vi "mohlat.vi"() -> ()   [LabVIEW 2017]
uses:
  <vilib>/Instr/_visa.llb/VISA Configure Serial Port (Instr).vi
  <vilib>/Utility/file.llb/Read Delimited Spreadsheet (string).vi
  <vilib>/Utility/file.llb/Write Delimited Spreadsheet (string).vi
panel:
  in  "pass":string="1234"
  out "number of users":i32
  in  "new pass":string caption="please enter new password"
  out "array w/ subset deleted":i32[](array[numeric])
  out "Array":i32[](array[numeric])
  out "subarray":string[][](array[string])
  out "min value":i32
  out "max value":i32
  out "SERIAL ID":string
  out "FULL NAME":string
  out "picture3":picture
  out "concatenated string":string
  out "appended array 4":string[](array[string])
  out "appended array 3":string[][](array[string])
  out "sabte tarikh":string[][](array[string])
  out "payam":string
  out "matrix of the data":string[][](array[string])
  in  "file path (text format)":path
  out "appended array 2":string[][](array[string])
  out "output array":string[](array[string])
  out "data base":string[][](array[string])
  out "appended array":string[](array[string])
  out "massage":string
  in  "Cluster":T1
  in  "Boolean":bool
  in  "Combo Box":string(combo)
  in  "password":bool
  in  "password:":string caption="enter password"
  out "PASSWORD MASSAGE":string
  out "error out":errorcluster
  in  "VISA resource name":refnum<visa-resource-name>
  out "read buffer":string
  in  "stop":bool
  in  "setting":bool
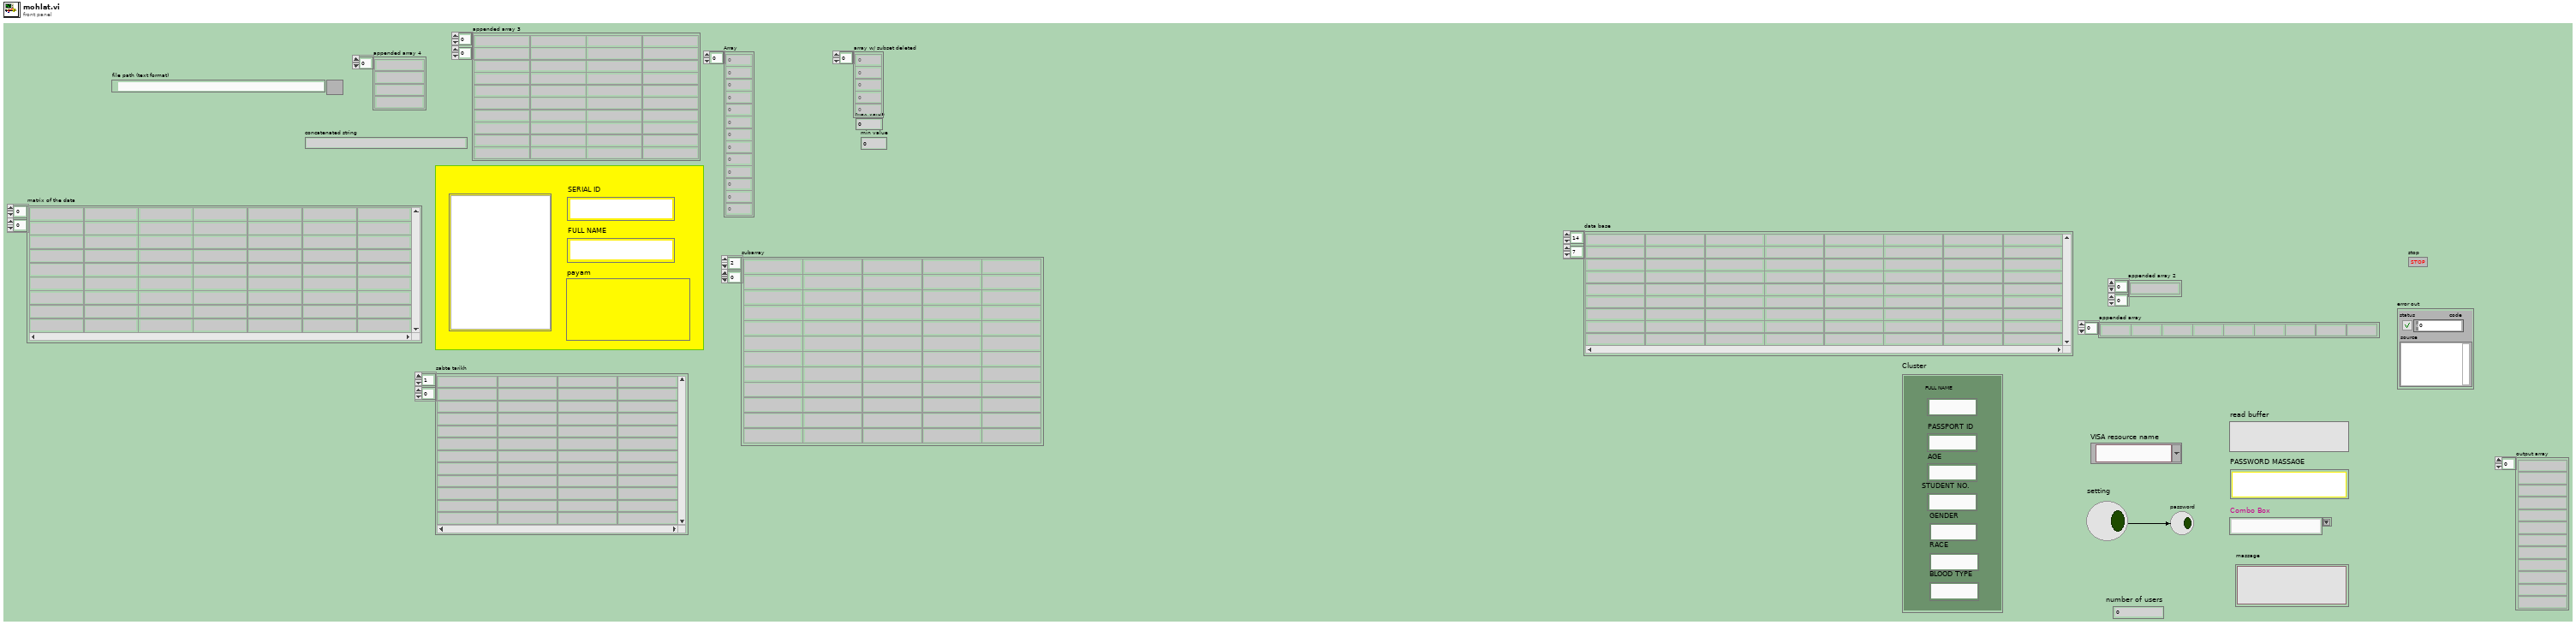
[diagram p1: front panel]
types:
  T1 = cluster{"FULL NAME":string, "PASSPORT ID":string, "AGE":string, "STUDENT NO.":string, "GENDER":string, "RACE":string, "BLOOD TYPE":string}
  T2 = cluster{"all rows[0]":string, "all rows[1]":string, "all rows[2]":string, "all rows[3]":string, "all rows[4]":string, "all rows[5]":string, "all rows[6]":string, "all rows[7]":string, "all rows[8]":string}
  T3 = typedef "imagedata.ctl" = cluster{"image type":i32, "image depth":i32, "image":u8[], "mask":u8[], "colors":u32[], "Rectangle":cluster{"left":i16, "top":i16, "right":i16, "bottom":i16}}
  T4 = cluster{string, string, string, string, string, string, string}
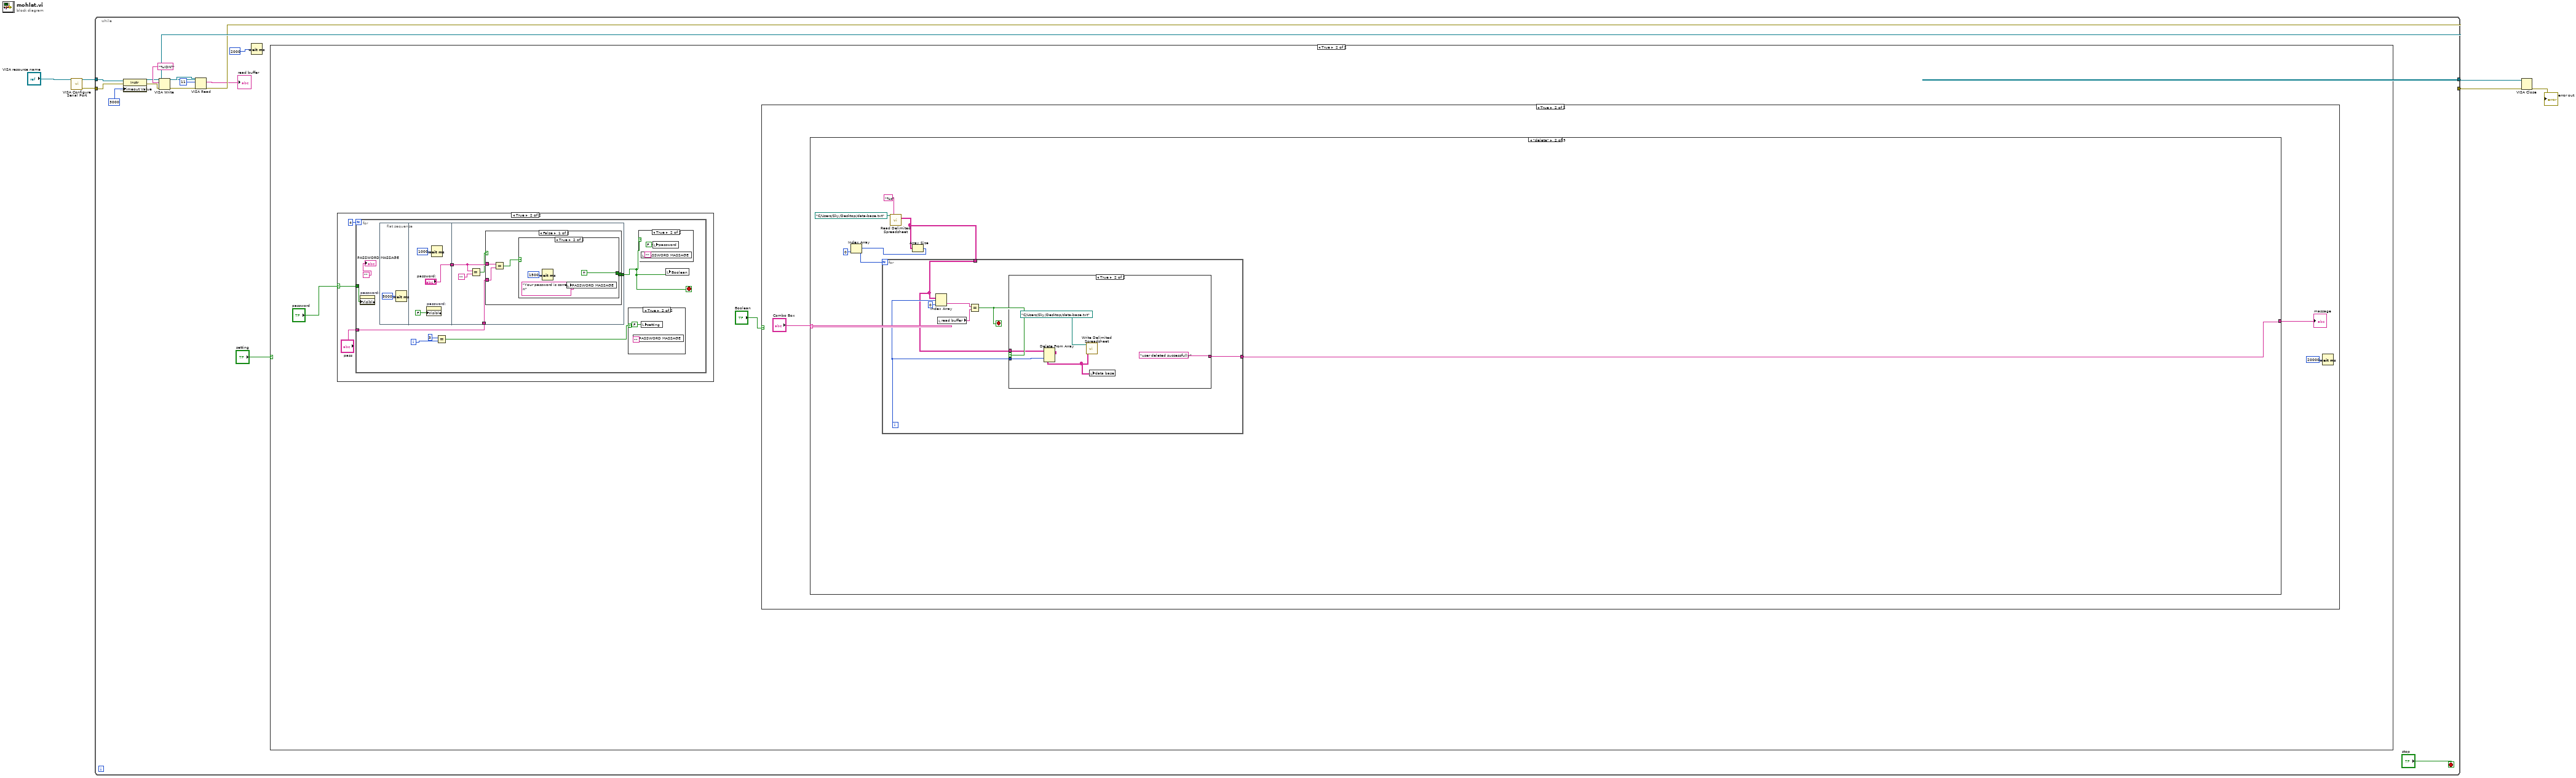
[diagram p0: block diagram]
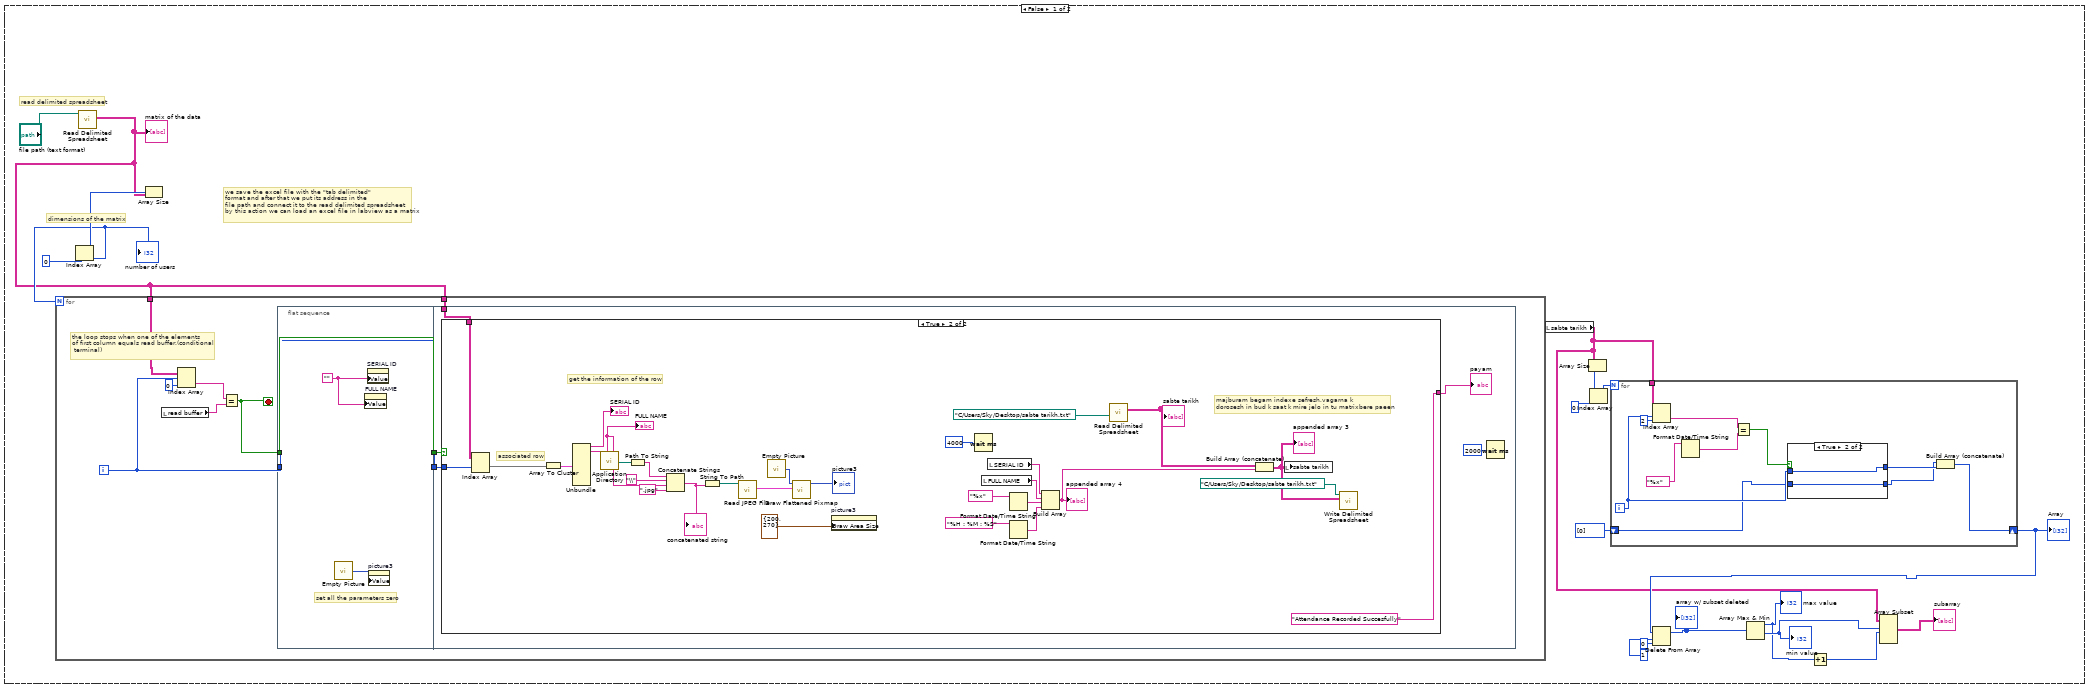
[diagram p2: hidden frame]
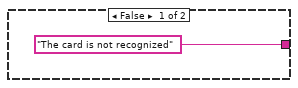
[diagram p4: hidden frame]
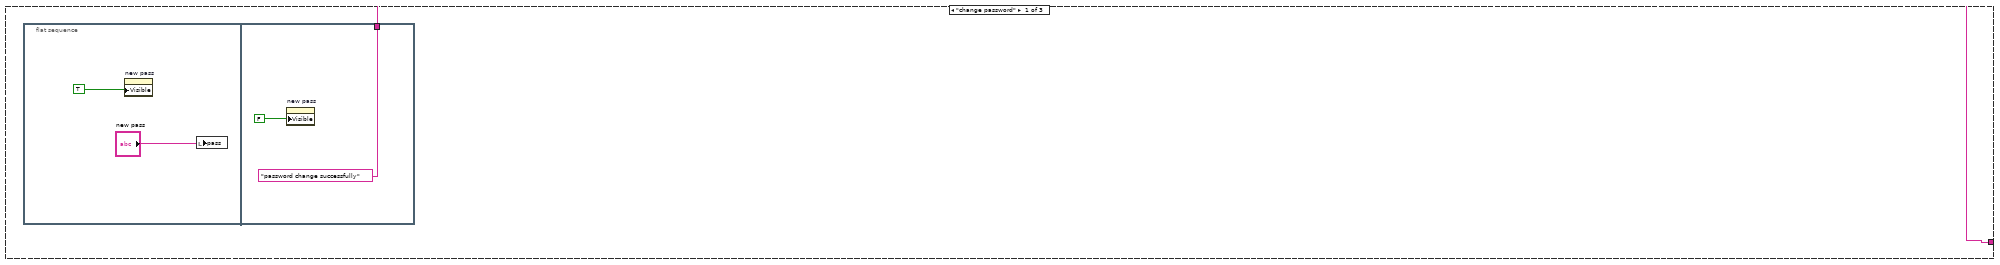
[diagram p6: hidden frame]
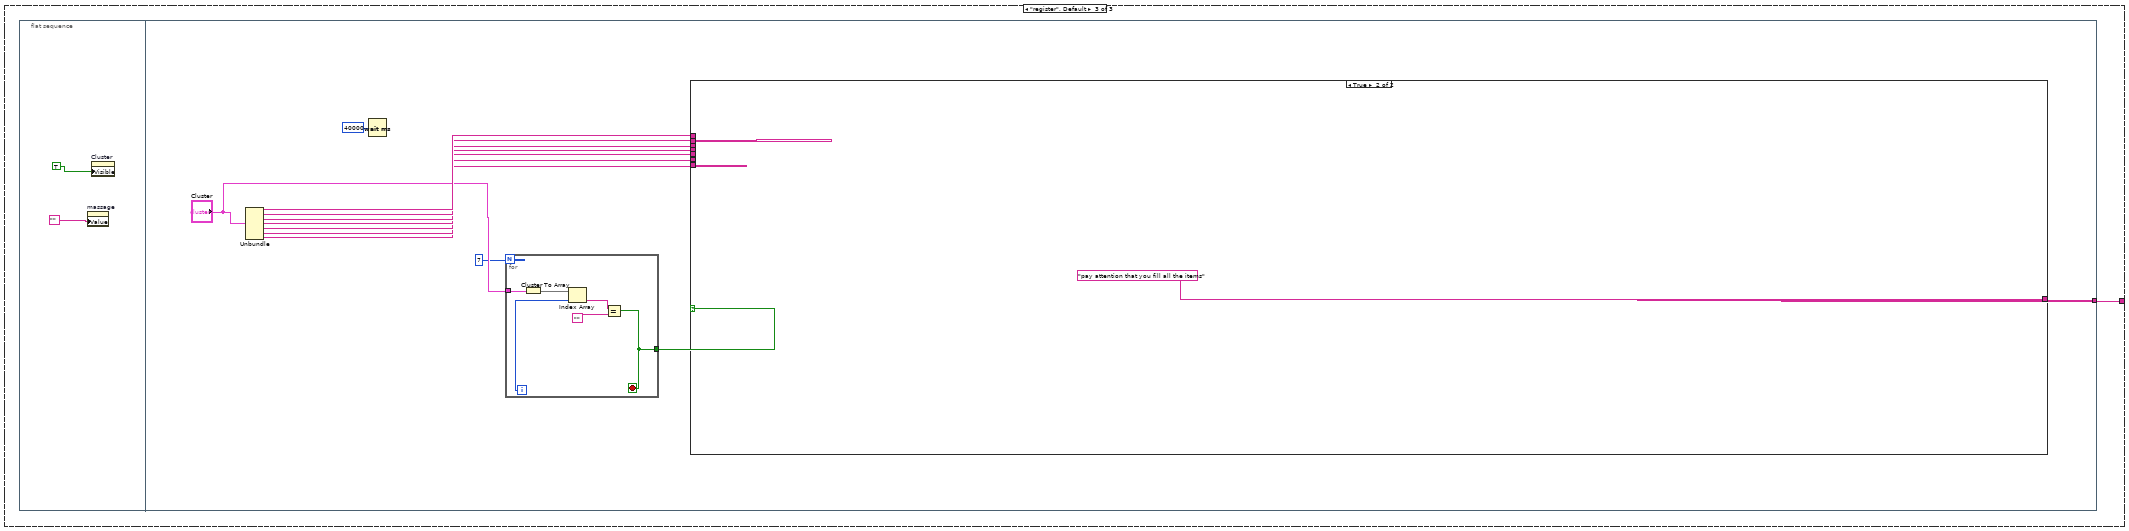
[diagram p8: hidden frame]
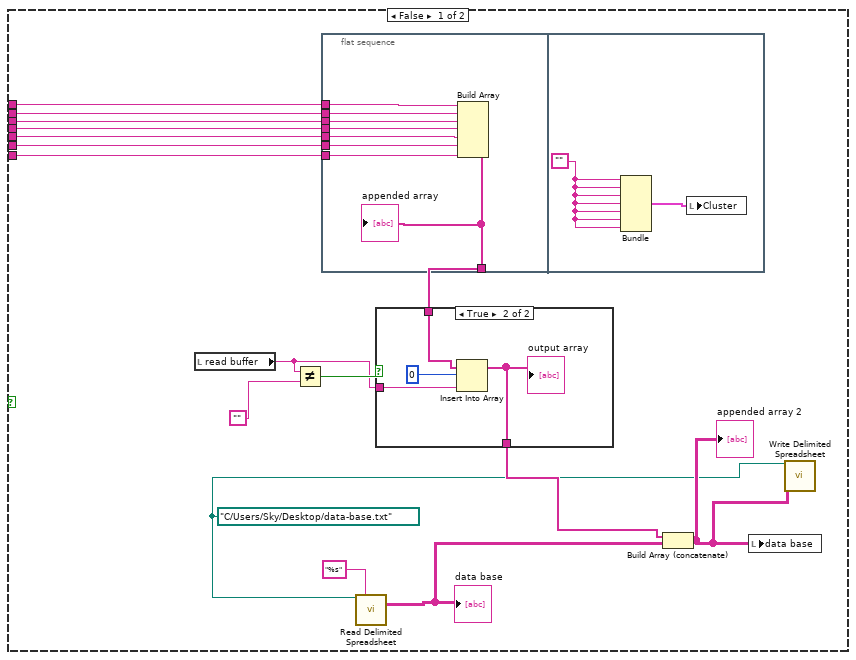
[diagram p9: hidden frame]
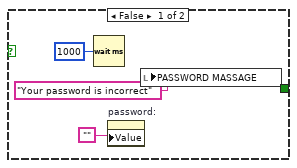
[diagram p14: hidden frame]
diagram:
  n1 = call-poly "VISA Configure Serial Port"("VISA resource name"="VISA resource name") -> ("VISA resource name out"=w5:refnum<visa-resource-name>, "error out"=w4:errorcluster)  [unwired: 13 in]
  n2 = while {
    tunnel: w5 -> [w14]
    tunnel: [w11] -> w2
    tunnel: w4 -> [w12]
    tunnel: [w10] -> w1
    stop <- "stop" stop-if-true
    n3 = property class="Instr"(reference=w14, error in=w12, "General Settings:Timeout Value"=u32 3000) -> (reference out=w17:refnum<visa-resource-name>, error out=w16:errorcluster)
    n4 = VISA Write(VISA resource name=w17, write buffer="%IDN?", error in (no error)=w16) -> (VISA resource name out=w15:refnum<visa-resource-name>, error out=w20:errorcluster)  [unwired: 1 out]
    n5 = VISA Read(VISA resource name=w15, byte count=u32 11, error in (no error)=w20) -> (VISA resource name out=w11:refnum<visa-resource-name>, read buffer=→"read buffer":string, error out=w10:errorcluster)  [unwired: 1 out]
    n6 = Wait (ms)(milliseconds to wait=u32 2000) -> ()  [unwired: 1 out]
    n7 = case shown="True" "setting" {
      frame False {
        # "dimensions of the matrix"
        # "read delimited spreadsheet"
        # "we save the excel file with the \"tab delimited\"\nformat and after that we put its address in the \nfile path and connect it to the read delimited spreadsheet \nby this action we can load an excel file in labview as a matrix"
        n8 = call-poly <vilib>:"Read Delimited Spreadsheet.vi"("file path (dialog if empty)"="file path (text format)") -> ("all rows"=w35:string[][])  [unwired: 9 in, 5 out]
        "matrix of the data" <- w35
        n9 = Array Size(array=w35) -> (size(s)=w38:i32[])
        n10 = Index Array(array=w38, index=0) -> (element=w36:i32)
        "number of users" <- w36
        n11 = for {
          N: w36 -> [_]
          tunnel: w35 -> [w58]
          tunnel: w35 -> [w53]
          i -> [w56]
          stop <- w57 stop-if-true
          # "the loop stops when one of the elements \nof first column equals read buffer.(conditional\n terminal)"
          n12 = local read "read buffer"() -> (w59:string)
          n13 = Index Array(array=w53, index (row)=w56, index (col)=0 ("disabled index (col)")) -> (element=w60:string)
          n14 = Equal?(x=w60, y=w59) -> (x = y?=w57:bool)
          n15 = flat-sequence {
            tunnel: w56 -> [w64]
            tunnel: w57 -> [w65]
            tunnel: [w65] -> w55
            tunnel: [w64] -> w54
            tunnel: w58 -> [w70]
            tunnel: w55 -> [w69]
            tunnel: w54 -> [w68]
            frame #0 {
              w62 = ""
              # "set all the parameters zero"
              n16 = call "Empty Picture"() -> ("empty picture"=w63:picture)
              n17 = property on="FULL NAME" class="Str"("Value"=w62) -> ()  [unwired: 2 in, 2 out]
              n18 = property on="SERIAL ID" class="Str"("Value"=w62) -> ()  [unwired: 2 in, 2 out]
              n19 = property on="picture3" class="Pict"("Value"=w63) -> ()  [unwired: 2 in, 2 out]
            }
            frame #1 {
              n20 = case shown="True" w69 {
                tunnel: w70 -> [_ w97]
                tunnel: w68 -> [_ w96]
                tunnel: ["The card is not recognized" ("format (%.3f)") "Attendance Recorded Succesfully" ("format (%.3f)")] -> w67
                frame False {
                }
                frame True {
                  # "majburam begam indexe sefresh,vagarna k \ndorosesh in bud k saat k mire jelo in tu matrixbere paeen"
                  # "get the information of the row"
                  # "associated row"
                  n21 = Index Array(array=w97, index (row)=w96) -> (element=w100:string[])  [unwired: 1 in]
                  n22 = Array To Cluster(array=w100) -> (cluster=w98:T2)
                  n23 = Unbundle(w98) -> ("all rows[0]"=→"SERIAL ID":string, "all rows[1]"=w83:string)  [unwired: 7 out]
                  "FULL NAME" <- w83
                  n24 = call <vilib>:"Application Directory.vi"() -> ("Application Directory"=w87:path)
                  n25 = Path To String(path=w87) -> (string=w88:string)
                  n26 = Concatenate Strings(w88, "\\" ("string"), w83, ".jpg" ("string")) -> (w85:string)
                  "concatenated string" <- w85
                  n27 = String To Path(string=w85) -> (path=w89:path)
                  n28 = call <vilib>:"Read JPEG File.vi"("path to JPEG file"=w89) -> ("image data"=w92:T3)  [unwired: 8 in, 2 out]
                  n29 = call "Empty Picture"() -> ("empty picture"=w90:picture)
                  n30 = call <vilib>:"Draw Flattened Pixmap.vi"("image data"=w92, "picture"=w90) -> ("new picture"=→"picture3":picture)  [unwired: 7 in]
                  n31 = property on="picture3" class="Pict"("Draw Area Size"=cluster{"Width":u32, "Height":u32} {"Width"=200, "Height"=270}) -> ()  [unwired: 2 in, 2 out]
                  n32 = Wait (ms)(milliseconds to wait=u32 4000) -> ()  [unwired: 1 out]
                  n33 = local read "FULL NAME"() -> (w78:string)
                  n34 = local read "SERIAL ID"() -> (w79:string)
                  n35 = Format Date/Time String(time format string (%c)="%x") -> (date/time string=w76:string)  [unwired: 2 in]
                  n36 = Format Date/Time String(time format string (%c)="%H : %M : %S") -> (date/time string=w75:string)  [unwired: 2 in]
                  n37 = Build Array(w79, w78, w76, w75) -> (w77:string[])
                  "appended array 4" <- w77
                  n38 = call-poly <vilib>:"Read Delimited Spreadsheet.vi"("file path (dialog if empty)"=path "C:/Users/Sky/Desktop/sabte tarikh.txt") -> ("all rows"=w73:string[][])  [unwired: 9 in, 5 out]
                  "sabte tarikh" <- w73
                  n39 = Build Array (concatenate)(w73, w77) -> (w72:string[][])
                  "appended array 3" <- w72
                  n40 = local write "sabte tarikh"(w72) -> ()
                  n41 = call-poly <vilib>:"Write Delimited Spreadsheet.vi"("file path (dialog if empty)"=path "C:/Users/Sky/Desktop/sabte tarikh.txt", "2D data"=w72) -> ()  [unwired: 12 in, 2 out]
                }
              }
              "payam" <- w67
              n42 = Wait (ms)(milliseconds to wait=u32 2000) -> ()  [unwired: 1 out]
            }
          }
        }
        n43 = local read "sabte tarikh"() -> (w23:string[][])
        n44 = Array Size(array=w23) -> (size(s)=w33:i32[])
        n45 = Index Array(array=w33, index=0) -> (element=w22:i32)
        n46 = for {
          N: w22 -> [_]
          tunnel: w23 -> [w48]
          shift-right: [w42] -> w27
          shift-left: i32[] [0] -> [w41]
          i -> [w44]
          n47 = Index Array(array=w48, index (row)=w44, index (col)=2) -> (element=w47:string)
          n48 = Format Date/Time String(time format string (%c)="%x") -> (date/time string=w46:string)  [unwired: 2 in]
          n49 = Equal?(x=w47, y=w46) -> (x = y?=w45:bool)
          n50 = case shown="True" w45 {
            tunnel: w44 -> [_ w52]
            tunnel: [_ w52] -> w43
            tunnel: w41 -> [_ w51]
            tunnel: [_ w51] -> w40
            frame False {
            }
            frame True {
            }
          }
          n51 = Build Array (concatenate)(w40, w43) -> (w42:i32[])
        }
        "Array" <- w27
        n52 = Delete From Array(array=w27, length=1, index=0) -> (array with subset deleted=w24:i32[])  [unwired: 1 out]
        "array w/ subset deleted" <- w24
        n53 = Array Max & Min(array=w24) -> (max value=w29:i32, min value=w30:i32)  [unwired: 2 out]
        "max value" <- w29
        "min value" <- w30
        n54 = Increment(x=w29) -> (x+1=w32:i32)
        n55 = Array Subset(array=w23, index (row)=w30, length (row)=w32) -> (→"subarray":string[][])  [unwired: 2 in]
      }
      frame True {
        n56 = case shown="True" "password" {
          selector: "password" -> [_ w183]
          frame False {
          }
          frame True {
            n57 = for {
              N: 4 -> [_]
              tunnel: "pass" -> [w192]
              tunnel: w183 -> [w187]
              i -> [w190]
              stop <- w185 stop-if-true
              n58 = property on="password:" class="Str"("Visible"=w187) -> ()  [unwired: 2 in, 2 out]
              n59 = flat-sequence {
                tunnel: ["password:"] -> w191
                tunnel: w191 -> [w203]
                tunnel: w192 -> [w205]
                tunnel: [w201] -> w185
                frame #0 {
                  n60 = Wait (ms)(milliseconds to wait=u32 5000) -> ()  [unwired: 1 out]
                }
                frame #1 {
                  n61 = property on="password:" class="Str"("Visible"=FALSE) -> ()  [unwired: 2 in, 2 out]
                  n62 = Wait (ms)(milliseconds to wait=u32 1000) -> ()  [unwired: 1 out]
                }
                frame #2 {
                  n63 = Equal?(x=w203, y="") -> (x = y?=w202:bool)
                  n64 = case shown="False" w202 {
                    tunnel: [w209 _] -> w201
                    tunnel: w205 -> [w208 _]
                    tunnel: w203 -> [w206 _]
                    frame False {
                      n65 = Equal?(x=w206, y=w208) -> (x = y?=w207:bool)
                      n66 = case shown="True" w207 {
                        tunnel: [_ TRUE] -> w209
                        frame False {
                          n67 = Wait (ms)(milliseconds to wait=u32 1000) -> ()  [unwired: 1 out]
                          n68 = property on="password:" class="Str"("Value"="") -> ()  [unwired: 2 in, 2 out]
                          n69 = local write "PASSWORD MASSAGE"("Your password is incorrect") -> ()
                        }
                        frame True {
                          n70 = Wait (ms)(milliseconds to wait=u32 1500) -> ()  [unwired: 1 out]
                          n71 = local write "PASSWORD MASSAGE"("Your password is correct\n") -> ()
                        }
                      }
                    }
                    frame True {
                    }
                  }
                }
              }
              n72 = Equal?(x=3, y=w190) -> (x = y?=w186:bool)
              n73 = case shown="True" w186 {
                frame False {
                }
                frame True {
                  n74 = local write "PASSWORD MASSAGE"("") -> ()
                  n75 = local write "setting"(FALSE) -> ()
                }
              }
              n76 = case shown="True" w185 {
                frame False {
                }
                frame True {
                  n77 = local write "PASSWORD MASSAGE"("") -> ()
                  n78 = local write "password"(FALSE) -> ()
                }
              }
              n79 = local write "Boolean"(w185) -> ()
              "PASSWORD MASSAGE" <- ""
            }
          }
        }
        n80 = case shown="True" "Boolean" {
          frame False {
          }
          frame True {
            n81 = case shown="\"delete\"" "Combo Box" {
              tunnel: [w106 w111 w130] -> w104
              frame "change password" {
                n82 = flat-sequence {
                  tunnel: ["password change successfully"] -> w106
                  frame #0 {
                    n83 = property on="new pass" class="Str"("Visible"=TRUE) -> ()  [unwired: 2 in, 2 out]
                    n84 = local write "pass"("new pass") -> ()
                  }
                  frame #1 {
                    n85 = property on="new pass" class="Str"("Visible"=FALSE) -> ()  [unwired: 2 in, 2 out]
                  }
                }
              }
              frame "delete" {
                n86 = call-poly <vilib>:"Read Delimited Spreadsheet.vi"("file path (dialog if empty)"=path "C:/Users/Sky/Desktop/data-base.txt", "format (%s)"="%s" ("format (%.3f)")) -> ("all rows"=w112:string[][])  [unwired: 8 in, 5 out]
                n87 = Array Size(array=w112) -> (size(s)=w117:i32[])
                n88 = Index Array(array=w117, index=0) -> (element=w114:i32)
                n89 = for {
                  N: w114 -> [_]
                  tunnel: [w119] -> w111
                  tunnel: w112 -> [w118]
                  i -> [w120]
                  stop <- w121 stop-if-true
                  n90 = Index Array(array=w118, index (row)=w120, index (col)=0 ("disabled index (col)")) -> (element=w123:string)
                  n91 = local read "read buffer"() -> (w122:string)
                  n92 = Equal?(x=w123, y=w122) -> (x = y?=w121:bool)
                  n93 = case shown="True" w121 {
                    tunnel: w118 -> [_ w129]
                    tunnel: w120 -> [_ w128]
                    tunnel: [_ "user deleted successfully"] -> w119
                    frame False {
                    }
                    frame True {
                      n94 = Delete From Array(array=w129, index (row)=w128) -> (array with subset deleted=w125:string[][])  [unwired: 2 in, 1 out]
                      n95 = call-poly <vilib>:"Write Delimited Spreadsheet.vi"("file path (dialog if empty)"=path "C:/Users/Sky/Desktop/data-base.txt", "2D data"=w125) -> ()  [unwired: 12 in, 2 out]
                      n96 = local write "data base"(w125) -> ()
                    }
                  }
                }
              }
              frame "register", Default {
                n97 = flat-sequence {
                  tunnel: [w135] -> w130
                  frame #0 {
                    n98 = property on="massage" class="Str"("Value"="") -> ()  [unwired: 2 in, 2 out]
                    n99 = property on="Cluster" class="Clust (strict)"("Visible"=TRUE) -> ()  [unwired: 2 in, 2 out]
                  }
                  frame #1 {
                    n100 = Unbundle("Cluster") -> ("FULL NAME"=w144:string, "PASSPORT ID"=w143:string, "AGE"=w142:string, "STUDENT NO."=w141:string, "GENDER"=w140:string, "RACE"=w139:string, "BLOOD TYPE"=w138:string)
                    n101 = Wait (ms)(milliseconds to wait=u32 40000) -> ()  [unwired: 1 out]
                    n102 = for {
                      N: 7 -> [_]
                      tunnel: "Cluster" -> [w181]
                      tunnel: [w176] -> w133
                      i -> [w179]
                      stop <- w176 stop-if-true
                      n103 = Cluster To Array(cluster=w181) -> (array=w180:string[])
                      n104 = Index Array(array=w180, index=w179) -> (element=w178:string)
                      n105 = Equal?(x=w178, y="") -> (x = y?=w176:bool)
                    }
                    n106 = case shown="True" w133 {
                      tunnel: [_ "pay attention that you fill all the items"] -> w135
                      tunnel: w144 -> [w159 _]
                      tunnel: w143 -> [w158 _]
                      tunnel: w142 -> [w157 _]
                      tunnel: w141 -> [w156 _]
                      tunnel: w140 -> [w155 _]
                      tunnel: w139 -> [w154 _]
                      tunnel: w138 -> [w153 _]
                      frame False {
                        w146 = path "C:/Users/Sky/Desktop/data-base.txt" ("file path (dialog if empty)")
                        n107 = local read "read buffer"() -> (w149:string)
                        n108 = Not Equal?(x=w149, y="") -> (x != y?=w151:bool)
                        n109 = flat-sequence {
                          tunnel: w159 -> [w172]
                          tunnel: w158 -> [w171]
                          tunnel: w157 -> [w170]
                          tunnel: w156 -> [w169]
                          tunnel: w155 -> [w168]
                          tunnel: w154 -> [w167]
                          tunnel: w153 -> [w166]
                          tunnel: [w165] -> w150
                          frame #0 {
                            n110 = Build Array(w172, w171, w170, w169, w168, w167, w166) -> (w165:string[])
                            "appended array" <- w165
                          }
                          frame #1 {
                            w173 = ""
                            n111 = Bundle(w173, w173, w173, w173, w173, w173, w173) -> (w174:T4)  [unwired: 1 in]
                            n112 = local write "Cluster"(w174) -> ()
                          }
                        }
                        n113 = call-poly <vilib>:"Read Delimited Spreadsheet.vi"("file path (dialog if empty)"=w146, "format (%s)"="%s" ("format (%.3f)")) -> ("all rows"=w145:string[][])  [unwired: 8 in, 5 out]
                        "data base" <- w145
                        n114 = case shown="True" w151 {
                          tunnel: w150 -> [_ w164]
                          tunnel: w149 -> [_ w163]
                          tunnel: [_ w161] -> w148
                          frame False {
                          }
                          frame True {
                            n115 = Insert Into Array(array=w164, index=0, new element=w163) -> (w161:string[])
                            "output array" <- w161
                          }
                        }
                        n116 = Build Array (concatenate)(w148, w145) -> (w147:string[][])
                        "appended array 2" <- w147
                        n117 = local write "data base"(w147) -> ()
                        n118 = call-poly <vilib>:"Write Delimited Spreadsheet.vi"("file path (dialog if empty)"=w146, "2D data"=w147) -> ()  [unwired: 12 in, 2 out]
                      }
                      frame True {
                      }
                    }
                  }
                }
              }
            }
            "massage" <- w104
            n119 = Wait (ms)(milliseconds to wait=u32 20000) -> ()  [unwired: 1 out]
          }
        }
      }
    }
  }
  n120 = VISA Close(VISA resource name=w2, error in (no error)=w1) -> (error out=→"error out":errorcluster)
